vi "Test Get Latest Broadcast Content Correct.vi"(8 "error in (no error)":errorcluster, 11 "Test Case In":refnum<class "Debugger Test.lvclass">) -> (0 "error out":errorcluster, 3 "Test Case Out":refnum<class "Debugger Test.lvclass">)   [LabVIEW 2020, in "Debugger Test.lvclass"]
uses:
  Debugger Test.lvclass
  Debugger Test.lvclass/Debugger Test.ctl
  source/Process/Debug Process.lvclass
  source/Debugger/Debugger.lvclass
  source/Debug Data/Debug Data.lvclass
  source/Debug Data/Raw Debug Data.ctl
  <vilib>/Astemes/Triarc Framework/Broadcast Event Helpers/Broadcast Event Helpers.lvlib
  770d5042-3263-43ff-84ad-3943cd9ed827.vi
  C:/Users/anton/Documents/GitHub/triarc-debugger/source/Process/Debug Process.lvclass
  C:/Users/anton/Documents/GitHub/triarc-debugger/source/Debugger/Debugger.lvclass
  C:/Users/anton/Documents/GitHub/triarc-debugger/source/Debug Data Event/Debug Data Listener.lvclass
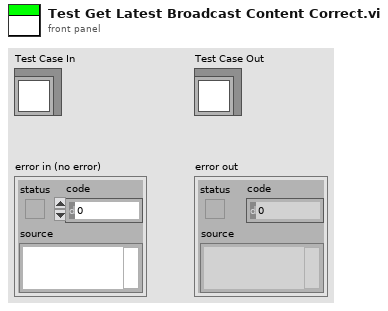
[diagram p1: front panel]
types:
  T1 = typedef "Debug Data.lvclass/Raw Debug Data.ctl" = cluster{"Action":string, "Call Chain":string, "Process":string, "Message":string, "Message Data":variant, "Time":dbl}
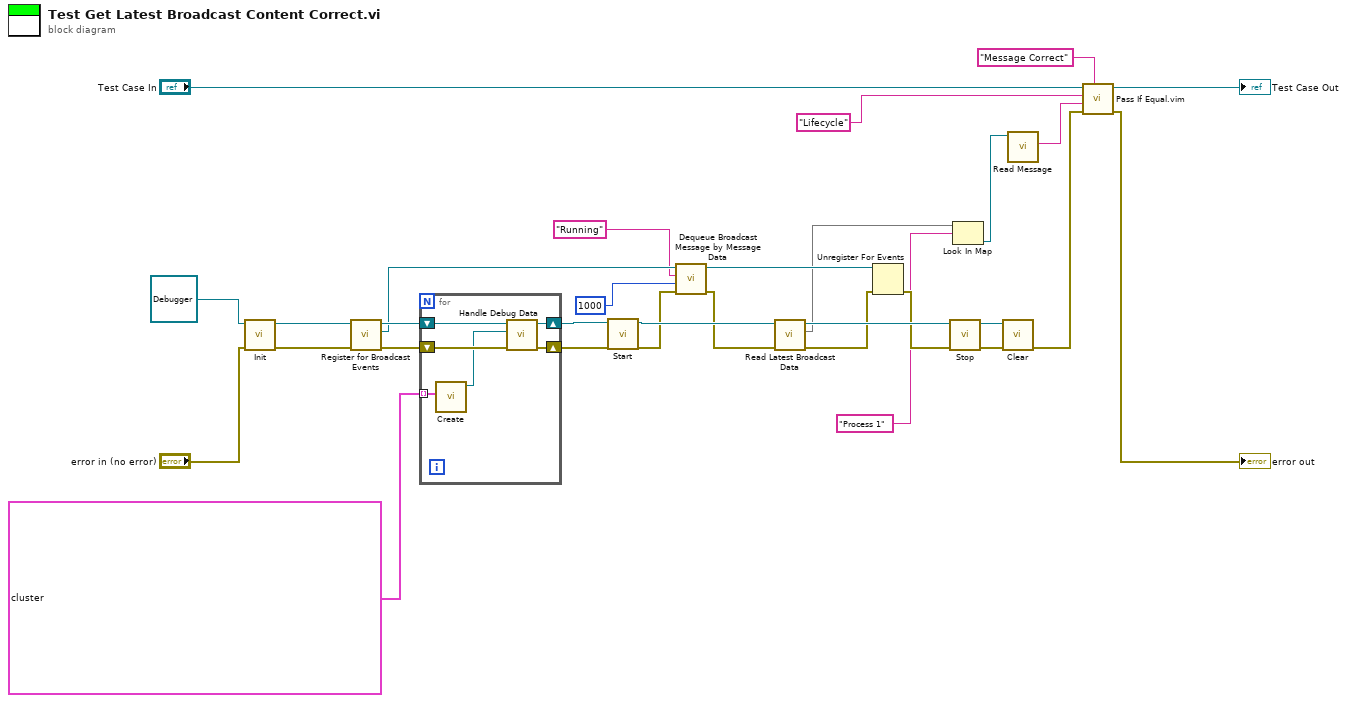
[diagram p0: block diagram]
diagram:
  n1 = call-dynamic "Init.vi"("error in (no error)"="error in (no error)", "Process In"=refnum<class "Debugger.lvclass"> refnum ("Debug Data Event In 2")) -> ("error out"=w10:errorcluster, "Process Out"=w11:refnum<class "Debugger.lvclass">)  [unwired: 8 in]
  n2 = call "Register for Broadcast Events.vi"("error in (no error)"=w10, "Process In"=w11) -> ("error out"=w28:errorcluster, "Event Registration Refnum Out"=w9:refnum<event-registration>, "Process Out"=w23:refnum<class "Debugger.lvclass">)  [unwired: 7 in]
  n3 = for {
    shift-right: [w35] -> w27
    shift-left: w28 -> [w37]
    shift-right: [w36] -> w13
    shift-left: w23 -> [w34]
    tunnel: T1[] [{"Action"="Send", "Call Chain"="Test.vi:123456", "Process"="Process 1", "Message"="Init", "Message Data"=variant, "Time"=0.0}, {"Action"="Broadcast", "Call Chain"="", "Process"="Process 1", "Message"="Lifecycle", "Message Data"=variant, "Time"=0.0}, {"Action"="Receive", "Call Chain"="TF.lvlib:Process.lvclass:Handle Messages.vi:1960001", "Process"="Process 1", "Message"="Start", "Message Data"=variant, "Time"=0.0}] ("Debug Data Cluster") -> [w33] mode=indexing
    n4 = call "Create.vi"("Debug Data Cluster"=w33) -> ("Debug Data out"=w32:refnum<class "Debug Data.lvclass">)  [unwired: 9 in, 1 out]
    n5 = call-dynamic "Handle Debug Data.vi"("error in (no error)"=w37, "Debug Data.lvclass"=w32, "Debug Data Event In"=w34) -> ("error out"=w35:errorcluster, "Debug Data Event Out"=w36:refnum<class "Debugger.lvclass">)  [unwired: 7 in]
  }
  n6 = call "Start.vi"("error in (no error)"=w27, "Process In"=w13) -> ("error out"=w7:errorcluster, "Process Out"=w12:refnum<class "Debugger.lvclass">)  [unwired: 7 in, 1 out]
  n7 = call <vilib>:"Dequeue Broadcast Message by Message Data.vi"("error in (no error)"=w7, "Timeout (-1)"=1000, "Message Data"="Running", "Event Registration Refnum"=w9) -> ("error out"=w6:errorcluster, "Event Registration Refnum Out"=w8:refnum<event-registration>)  [unwired: 3 in, 3 out]
  n8 = call "Read Latest Broadcast Data.vi"("error in (no error)"=w6, "Debugger In"=w12) -> ("error out"=w18:errorcluster, "Latest Messages"=w3:map{string, refnum<class "Debug Data.lvclass">}, "Debugger Out"=w26:refnum<class "Debugger.lvclass">)  [unwired: 7 in]
  n9 = Unregister For Events(event registration refnum=w8, error in=w18) -> (error out=w17:errorcluster)
  n10 = call "Stop.vi"("error in (no error)"=w17, "Process In"=w26) -> ("error out"=w24:errorcluster, "Process Out"=w25:refnum<class "Debugger.lvclass">)  [unwired: 7 in, 1 out]
  n11 = Look In Map(map=w3, key="Process 1") -> (value=w16:refnum<class "Debug Data.lvclass">)  [unwired: 1 in, 1 out]
  n12 = call-dynamic "Clear.vi"("error in (no error)"=w24, "Process In"=w25) -> ("error out"=w20:errorcluster)  [unwired: 9 in]
  n13 = call "Read Message.vi"("Debug Data in"=w16) -> ("Message"=w2:string)  [unwired: 8 in, 2 out]
  n14 = call "Pass If Equal.vim"("Description"="Message Correct", "error in (no error)"=w20, "Actual"=w2, "Expected"="Lifecycle", "LUnit Test Case In"="Test Case In") -> ("error out"=→"error out":errorcluster, "LUnit Test Case Out"=→"Test Case Out":refnum<class "Debugger Test.lvclass">)  [unwired: 5 in]
